vi "BRig_dataExp_FPGA_count2ms.vi"() -> (2 "output_FPGA_count2ms":i32)   [LabVIEW 2014]
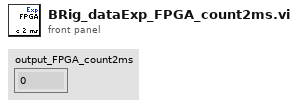
[diagram p1: front panel]
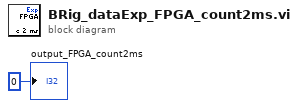
[diagram p0: block diagram]
diagram:
  "output_FPGA_count2ms" <- 0 ("output_iBlock")
